vi "TSM SSC Digital Write Static.vi"(0 "Digital TSM in":T1, 5 "State":T3 items=["0"=0, "1"=1, "X"=5], 11 "error in":errorcluster) -> (4 "Digital TSM out":T1, 15 "error out":errorcluster)   [LabVIEW 2020]
doc: "Writes a static state to all specified pin(s) and pin group(s). The selected pins remain in the specified state until the next pattern burst or call to this VI. If there are uncommitted changes to levels or the termination mode, this VI commits the changes to the pins.\n\nThis VI does not change the selected pin function. If you write a static state to a pin that does not have the Digital function selected, the new static state is stored by the digital pattern instrument, and affects the state of the pin the next time you change the selected function to Digital."
uses:
  <instrlib>/niDigital/niDigital.llb/niDigital Write Static Pin State.ctl
  TSM/TSM SSC Digital.ctl
  <vilib>/NI_TestStand_SemiconductorModule/NI_TestStand_Semiconductor_Module.lvlibp/PinMap/Digital Pattern/PinQueryContext/DigitalPatternPinQueryContext.lvclass
  SSC Digital/SSC Digital.ctl
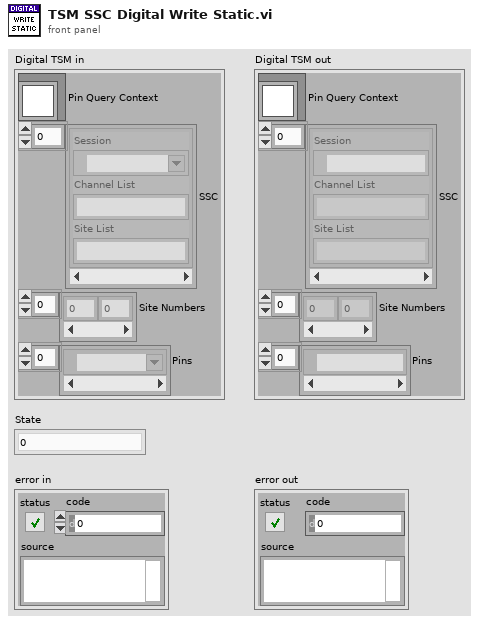
[diagram p1: front panel]
types:
  T1 = typedef "TSM SSC Digital.ctl" = cluster{"Pin Query Context":refnum<class "DigitalPatternPinQueryContext.lvclass">, "SSC":T2[], "Site Numbers":i32[], "Pins":tag[]}
  T2 = typedef "SSC Digital.ctl" = cluster{"Session":refnum<k15>, "Channel List":string, "Site List":string}
  T3 = typedef "niDigital Write Static Pin State.ctl" = u8
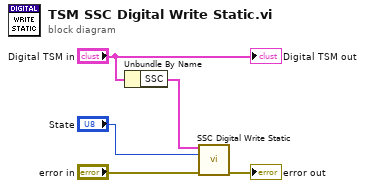
[diagram p0: block diagram]
diagram:
  n1 = Unbundle By Name("Digital TSM in") -> ("SSC"=w2:T2[])
  n2 = call "SSC Digital Write Static.vi"("Digital SSC in"=w2, "State"="State", "error in"="error in") -> ("error out"=→"error out":errorcluster)  [unwired: 11 in, 1 out]
  "Digital TSM out" <- "Digital TSM in"
